vi "Set Default Scalar and Offset.vi"(8 "error in (no error)":errorcluster, 10 "Calibration Type":string, 11 "Cree Communications in":refnum<class "Cree Communications.lvclass">) -> (0 "error out":errorcluster)   [LabVIEW 2015, in "Calibration.lvclass"]
uses:
  Calibration.lvclass
  Classes/Cree Communications/Class/Cree Communications.lvclass
  Classes/Cree Communications/Cree Comms Messages/Set Vsec Offset/Set Vsec Offset.lvclass
  Classes/Cree Communications/Cree Comms Messages/Set Vsec Scalar/Set Vsec Scalar.lvclass
  Classes/Cree Communications/Cree Comms Messages/Set String Current Offset/Set String Current Offset.lvclass
  Classes/Cree Communications/Cree Comms Messages/Set String Current Scalar/Set String Current Scalar.lvclass
  Classes/Cree Communications/Cree Comms Messages/Set ITemp Scalar/Set ITemp Scalar.lvclass
  Classes/Cree Communications/Cree Comms Messages/Set ITemp Offset/Set ITemp Offset.lvclass
  Classes/Cree Communications/Cree Comms Messages/CC Message/CC Message.lvclass/CC Message.ctl
  Classes/Cree Communications/Cree Comms Messages/CC Message/CC Message.lvclass
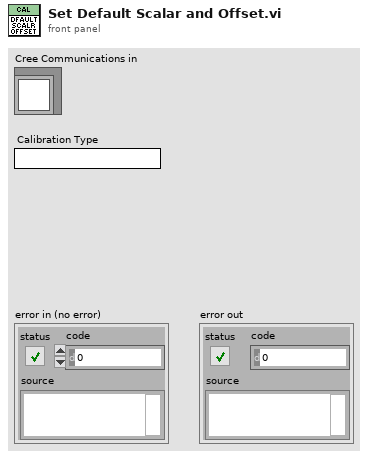
[diagram p1: front panel]
types:
  T1 = cluster{"Offset":dbl, "String":enum16{"Red", "BSY1", "BSY2"}}
  T2 = cluster{"Scalar":dbl, "String":enum16{"Red", "BSY1", "BSY2"}}
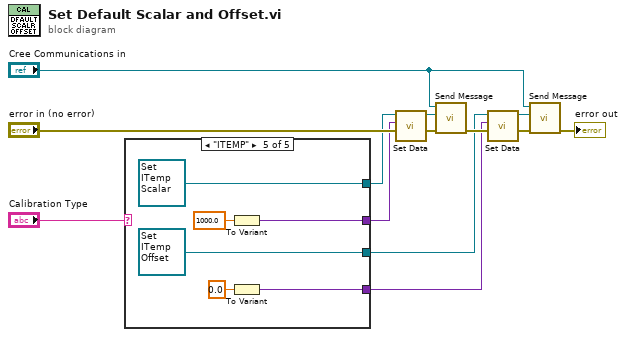
[diagram p0: block diagram]
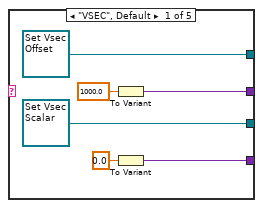
[diagram p2: hidden frame]
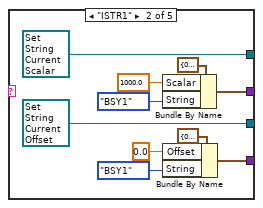
[diagram p3: hidden frame]
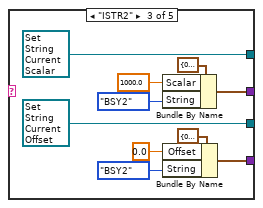
[diagram p4: hidden frame]
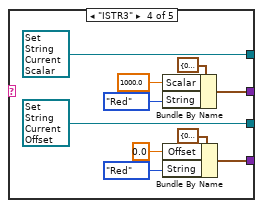
[diagram p5: hidden frame]
diagram:
  n1 = case shown="\"ITEMP\"" "Calibration Type" {
    tunnel: [refnum<class "Set Vsec Scalar.lvclass"> refnum ("Cree Comms Messages.lvlib:Set Vsec Scalar.lvclass") refnum<class "Set String Current Offset.lvclass"> refnum ("Cree Comms Messages.lvlib:Set String Current Offset.lvclass") refnum<class "Set String Current Offset.lvclass"> refnum ("Cree Comms Messages.lvlib:Set String Current Offset.lvclass") refnum<class "Set String Current Offset.lvclass"> refnum ("Cree Comms Messages.lvlib:Set String Current Offset.lvclass") refnum<class "Set ITemp Offset.lvclass"> refnum ("Cree Comms Messages.lvlib:Set ITemp Offset.lvclass")] -> w6
    tunnel: [w12 w23 w33 w43 w50] -> w5
    tunnel: [w13 w25 w35 w45 w51] -> w4
    tunnel: [refnum<class "Set Vsec Offset.lvclass"> refnum ("Cree Comms Messages.lvlib:Set Vsec Offset.lvclass") refnum<class "Set String Current Scalar.lvclass"> refnum ("Cree Comms Messages.lvlib:Set String Current Scalar.lvclass") refnum<class "Set String Current Scalar.lvclass"> refnum ("Cree Comms Messages.lvlib:Set String Current Scalar.lvclass") refnum<class "Set String Current Scalar.lvclass"> refnum ("Cree Comms Messages.lvlib:Set String Current Scalar.lvclass") refnum<class "Set ITemp Scalar.lvclass"> refnum ("Cree Comms Messages.lvlib:Set ITemp Scalar.lvclass")] -> w2
    frame "VSEC", Default {
      n2 = To Variant(anything=1000.0 ("Position 2")) -> (Variant=w13:variant)
      n3 = To Variant(anything=0.0 ("Position 2")) -> (Variant=w12:variant)
    }
    frame "ISTR1" {
      n4 = Bundle By Name(cluster=T2 {"Scalar"=0.0, "String"=enum."Red"} ("Message Type"), "Scalar"=1000.0 ("Position 2"), "String"=enum16{"Red", "BSY1", "BSY2"}."BSY1") -> (w25:T2)
      n5 = Bundle By Name(cluster=T1 {"Offset"=0.0, "String"=enum."Red"} ("Message Type"), "Offset"=0.0 ("Position 2"), "String"=enum16{"Red", "BSY1", "BSY2"}."BSY1") -> (w23:T1)
    }
    frame "ISTR2" {
      n6 = Bundle By Name(cluster=T2 {"Scalar"=0.0, "String"=enum."Red"} ("Message Type"), "Scalar"=1000.0 ("Position 2"), "String"=enum16{"Red", "BSY1", "BSY2"}."BSY2") -> (w35:T2)
      n7 = Bundle By Name(cluster=T1 {"Offset"=0.0, "String"=enum."Red"} ("Message Type"), "Offset"=0.0 ("Position 2"), "String"=enum16{"Red", "BSY1", "BSY2"}."BSY2") -> (w33:T1)
    }
    frame "ISTR3" {
      n8 = Bundle By Name(cluster=T2 {"Scalar"=0.0, "String"=enum."Red"} ("Message Type"), "Scalar"=1000.0 ("Position 2"), "String"=enum16{"Red", "BSY1", "BSY2"}."Red") -> (w45:T2)
      n9 = Bundle By Name(cluster=T1 {"Offset"=0.0, "String"=enum."Red"} ("Message Type"), "Offset"=0.0 ("Position 2"), "String"=enum16{"Red", "BSY1", "BSY2"}."Red") -> (w43:T1)
    }
    frame "ITEMP" {
      n10 = To Variant(anything=1000.0 ("Position 2")) -> (Variant=w51:variant)
      n11 = To Variant(anything=0.0 ("Position 2")) -> (Variant=w50:variant)
    }
  }
  n12 = call "Set Data.vi"("Data"=w4, "CC Message in"=w2) -> ("CC Message out"=w3:refnum<class "CC Message.lvclass">)  [unwired: 8 in, 1 out]
  n13 = call "Send Message.vi"("error in (no error)"="error in (no error)", "Cree Comms Message"=w3, "Acrobat Template in"="Cree Communications in") -> ("error out"=w8:errorcluster)  [unwired: 7 in, 1 out]
  n14 = call "Set Data.vi"("Data"=w5, "CC Message in"=w6) -> ("CC Message out"=w10:refnum<class "CC Message.lvclass">)  [unwired: 8 in, 1 out]
  n15 = call "Send Message.vi"("error in (no error)"=w8, "Cree Comms Message"=w10, "Acrobat Template in"="Cree Communications in") -> ("error out"=→"error out":errorcluster)  [unwired: 7 in, 1 out]
